vi "Open Child.vi"(8 "error in (no error)":errorcluster, 11 "Websocket Server in":refnum<class "Websocket Server.lvclass">) -> (0 "error out":errorcluster, 3 "Websocket Server out":refnum<class "Websocket Server.lvclass">)   [LabVIEW 2020, in "Stream-Websocket.lvlib" / "Websocket Server.lvclass"]
uses:
  Websocket Server.lvclass
  Websocket Server.lvclass/Websocket Server.ctl
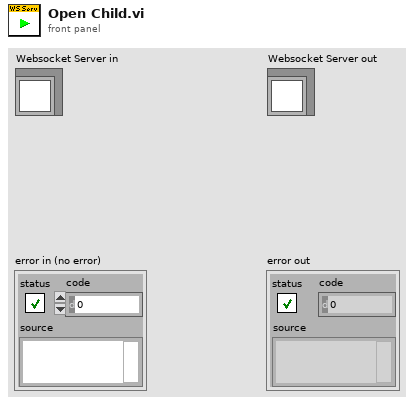
[diagram p1: front panel]
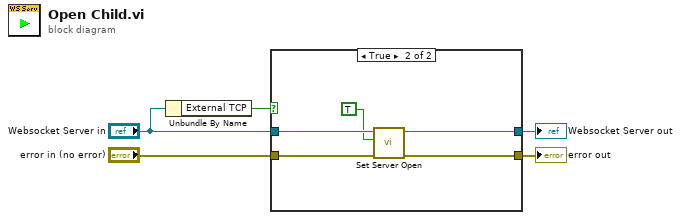
[diagram p0: block diagram]
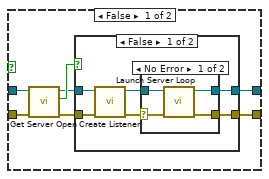
[diagram p2: hidden frame]
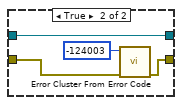
[diagram p4: hidden frame]
diagram:
  n1 = Unbundle By Name("Websocket Server in") -> ("External TCP"=w1:bool)
  n2 = case shown="True" w1 {
    tunnel: "error in (no error)" -> [w12 w32]
    tunnel: [w8 w30] -> w4
    tunnel: [w7 w29] -> w3
    tunnel: "Websocket Server in" -> [w6 w33]
    frame False {
      n3 = call "Get Server Open.vi"("error in (no error)"=w12, "Websocket Server in"=w6) -> ("error out"=w9:errorcluster, "Server Open"=w11:bool, "Websocket Server out"=w10:refnum<class "Websocket Server.lvclass">)  [unwired: 7 in]
      n4 = case shown="False" w11 {
        tunnel: w10 -> [w18 w28]
        tunnel: w9 -> [w17 w25]
        tunnel: [w14 w28] -> w8
        tunnel: [w13 w26] -> w7
        frame False {
          n5 = call "Create Listener.vi"("error in (no error)"=w17, "Websocket Server in"=w18) -> ("error out"=w16:errorcluster, "Websocket Server out"=w15:refnum<class "Websocket Server.lvclass">)  [unwired: 8 in]
          n6 = case shown="No Error" w16 {
            selector: w16 -> [w21 w23]
            tunnel: w15 -> [w22 w24]
            tunnel: [w20 w24] -> w14
            tunnel: [w19 w23] -> w13
            frame No Error {
              n7 = call "Launch Server Loop.vi"("error in (no error)"=w21, "Websocket Server in"=w22) -> ("error out"=w19:errorcluster, "Websocket Server out"=w20:refnum<class "Websocket Server.lvclass">)  [unwired: 8 in]
            }
            frame Error {
            }
          }
        }
        frame True {
          n8 = call <vilib>:"Error Cluster From Error Code.vi"("error in (no error)"=w25, "error code (0)"=-124003) -> ("error out"=w26:errorcluster)  [unwired: 7 in]
        }
      }
    }
    frame True {
      n9 = call "Set Server Open.vi"("error in (no error)"=w32, "Server Open"=TRUE, "Websocket Server in"=w33) -> ("error out"=w29:errorcluster, "Websocket Server out"=w30:refnum<class "Websocket Server.lvclass">)  [unwired: 7 in]
    }
  }
  "error out" <- w3
  "Websocket Server out" <- w4
